vi "Read from File.vi"(7 "Section Name":string, 8 "error in (no error)":errorcluster, 10 "INI Ref":T1, 11 "String Assertion in":refnum<class "String Assertion.lvclass">) -> (0 "error out":errorcluster, 2 "INI Ref out":T1, 3 "String Assertion out":refnum<class "String Assertion.lvclass">)   [LabVIEW 2020, in "MacroAssert.lvlib" / "String Assertion.lvclass"]
doc: "Reads associated parameters from the file identified by <B>INI Ref</B>."
uses:
  String Assertion.lvclass
  <vilib>/Utility/config.llb/Config Data RefNum.ctl
  String Assertion Type.ctl
  String Comparator.ctl
  <vilib>/Utility/error.llb/Error Cluster From Error Code.vi
  <vilib>/Utility/config.llb/Read Key (String).vi
  <vilib>/Utility/config.llb/Read Key (Boolean).vi
  Assertion Step/Assertion Step.lvclass
  SubVIs/Custom Errors/Custom Errors.lvlib
  <vilib>/Utility/config.llb/NI_LVConfig.lvlib
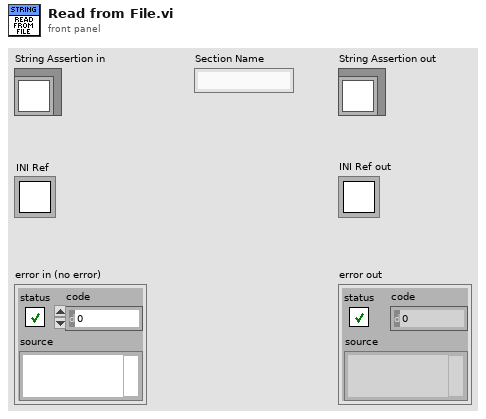
[diagram p1: front panel]
types:
  T1 = typedef "NI_LVConfig.lvlib/Config Data RefNum.ctl" = refnum<k1>
  T2 = typedef "MacroAssert.lvlib/String Assertion.lvclass/String Assertion Type.ctl" = enum16{"String Ctl Value", "Ctl Caption Property", "Ctl Tip Strip Property", "Frontmost VI Name", "Frontmost Window Name"}
  T3 = typedef "MacroAssert.lvlib/String Assertion.lvclass/String Comparator.ctl" = enum16{"Contains", "Equals", "Starts with", "Ends with", "Does not contain", "Does not equal"}
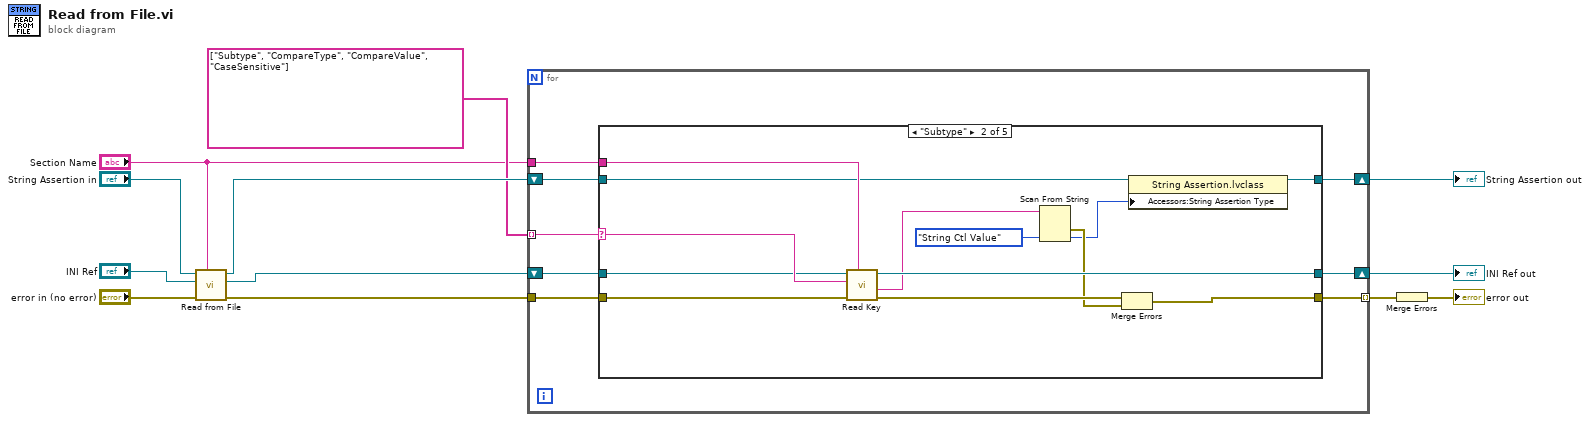
[diagram p0: block diagram]
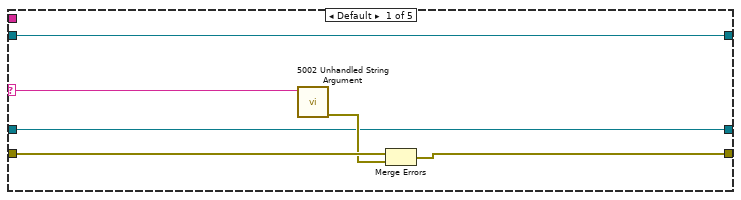
[diagram p2: hidden frame]
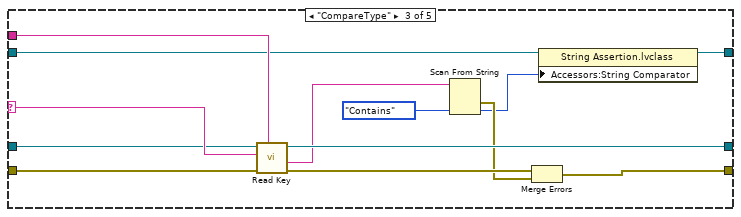
[diagram p3: hidden frame]
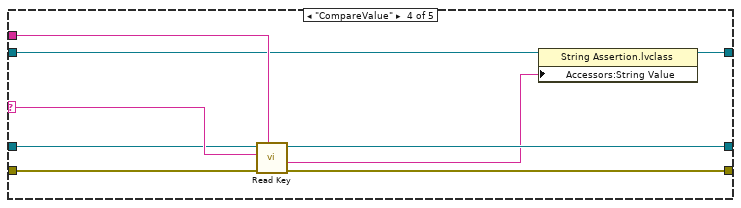
[diagram p4: hidden frame]
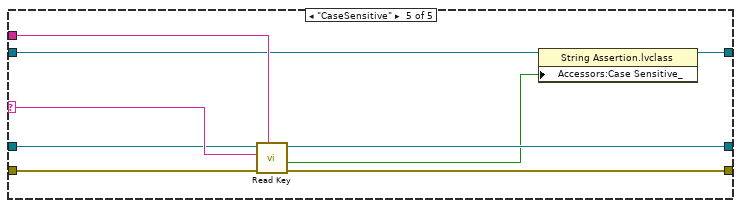
[diagram p5: hidden frame]
diagram:
  n1 = call-parent "Read from File.vi"("Section Name"="Section Name", "error in (no error)"="error in (no error)", "INI Ref"="INI Ref", "Assertion Step in"="String Assertion in") -> ("error out"=w10:errorcluster, "INI Ref out"=w9:T1, "Assertion Step out"=w12:refnum<class "String Assertion.lvclass">)  [unwired: 5 in]
  n2 = for {
    tunnel: string[] ["Subtype", "CompareType", "CompareValue", "CaseSensitive"] -> [w20] mode=indexing
    tunnel: w10 -> [w19]
    tunnel: "Section Name" -> [w18]
    shift-right: [w16] -> w2
    shift-left: w12 -> [w17]
    tunnel: [w15] -> w8 mode=indexing
    shift-right: [w13] -> w3
    shift-left: w9 -> [w14]
    n3 = case shown="\"Subtype\"" w20 {
      selector: w20 -> [w23 w34 w47 w56 w65]
      tunnel: w19 -> [w25 w39 w52 w61 w70]
      tunnel: w18 -> [_ w38 w51 w60 w69]
      tunnel: w17 -> [w26 w37 w50 w59 w68]
      tunnel: [w26 w36 w49 w58 w67] -> w16
      tunnel: [w22 w30 w43 w57 w66] -> w15
      tunnel: w14 -> [w21 w33 w46 w55 w64]
      tunnel: [w21 w32 w45 w54 w63] -> w13
      frame Default {
        n4 = call "5002 Unhandled String Argument.vi"("Argument"=w23) -> ("error out"=w24:errorcluster)  [unwired: 10 in]
        n5 = Merge Errors(w25, w24) -> (w22:errorcluster)
      }
      frame "Subtype" {
        n6 = call-poly <vilib>:"Read Key.vi"("section"=w38, "error in (no error)"=w39, "key"=w34, "refnum"=w33) -> ("error out"=w35:errorcluster, "value"=w31:string, "refnum out"=w32:T1)  [unwired: 4 in, 1 out]
        n7 = Scan From String(input string=w31, default 1=String_Assertion_Type."String Ctl Value" ("String Assertion Type")) -> (error out=w29:errorcluster, output 1=w28:T2)  [unwired: 3 in, 2 out]
        n8 = Merge Errors(w35, w29) -> (w30:errorcluster)
        n9 = property class="String Assertion.lvclass"(reference=w37, "Accessors:String Assertion Type"=w28) -> (reference out=w36:refnum<class "String Assertion.lvclass">)  [unwired: 1 in, 1 out]
      }
      frame "CompareType" {
        n10 = call-poly <vilib>:"Read Key.vi"("section"=w51, "error in (no error)"=w52, "key"=w47, "refnum"=w46) -> ("error out"=w48:errorcluster, "value"=w44:string, "refnum out"=w45:T1)  [unwired: 4 in, 1 out]
        n11 = Scan From String(input string=w44, default 1=String_Comparator."Contains" ("String Comparator")) -> (error out=w42:errorcluster, output 1=w41:T3)  [unwired: 3 in, 2 out]
        n12 = Merge Errors(w48, w42) -> (w43:errorcluster)
        n13 = property class="String Assertion.lvclass"(reference=w50, "Accessors:String Comparator"=w41) -> (reference out=w49:refnum<class "String Assertion.lvclass">)  [unwired: 1 in, 1 out]
      }
      frame "CompareValue" {
        n14 = call-poly <vilib>:"Read Key.vi"("section"=w60, "error in (no error)"=w61, "key"=w56, "refnum"=w55) -> ("error out"=w57:errorcluster, "value"=w53:string, "refnum out"=w54:T1)  [unwired: 4 in, 1 out]
        n15 = property class="String Assertion.lvclass"(reference=w59, "Accessors:String Value"=w53) -> (reference out=w58:refnum<class "String Assertion.lvclass">)  [unwired: 1 in, 1 out]
      }
      frame "CaseSensitive" {
        n16 = call-poly <vilib>:"Read Key.vi"("section"=w69, "error in (no error)"=w70, "key"=w65, "refnum"=w64) -> ("error out"=w66:errorcluster, "value"=w62:bool, "refnum out"=w63:T1)  [unwired: 4 in, 1 out]
        n17 = property class="String Assertion.lvclass"(reference=w68, "Accessors:Case Sensitive_"=w62) -> (reference out=w67:refnum<class "String Assertion.lvclass">)  [unwired: 1 in, 1 out]
      }
    }
  }
  "String Assertion out" <- w2
  "INI Ref out" <- w3
  n18 = Merge Errors(w8) -> (→"error out":errorcluster)
